vi "Read Key (Variant)__ogtk.vi"(5 "format string (%;%f)":string="%f", 7 "section":string, 8 "error in (no error)":errorcluster, 9 "type":variant, 10 "key (optional)":string, 11 "refnum":T1) -> (0 "error out":errorcluster, 1 "key-value":variant, 2 "found?":bool, 3 "refnum out":T1)   [LabVIEW 2017]
doc: "Reads a value associated with key in a specified section of the configuration data identified by refnum. If \"key\" input is not specified, the name of the variant object is used as the key. the \"found?\" output will be TRUE for compount objects (clusters) only if all elements (recursively) are found.\n\nFor example a Boolean named \"Enable\" with a value of TRUE would correspond to the key-value pair:\n\nEnable=TRUE\n\nNote: Special characters in section and key names will be escape-coded. These include the following: \\00-\\1F (non-printable chars); \"[\", \"]\", and \"=\" (INI syntax elements); \\FE (\"þ\") and \\FF (\"ÿ\") (legacy bracket encoding); Additionally, the escape character, \"\\\", will be escaped as \"\\\\\"."
uses:
  <vilib>/Utility/config.llb/Config Data RefNum.ctl
  <vilib>/Utility/config.llb/Read Key (String).vi
  <vilib>/Utility/config.llb/Read Key (Path).vi
  <vilib>/Utility/config.llb/Read Key (Boolean).vi
  <vilib>/Utility/config.llb/Read Key (Double).vi
  <vilib>/Utility/config.llb/Read Key (U32).vi
  <vilib>/Utility/config.llb/Read Key (I32).vi
  <vilib>/Utility/config.llb/NI_LVConfig.lvlib
panel:
  in  "Ref for recursive call":refnum<vi>
  # "Read Key (Variant).vi\n\nReads a variant key-value from INI file.\n\nPlease visit http://www.OpenG.org to learn about the\nOpen Source LabVIEW software movement.\n\nNOTICE -- YOU MUST LEAVE THIS NOTICE IN PLACE.  PER THE TERMS OF THE LICENSE BELOW, YOU MAY SUBLICENSE THIS SOFTWARE \nIN ANY WAY THAT DOES NOT CONFLICT WITH THIS LICENSE.\n\n### BSD License (http://www.opensource.org/licenses/bsd-license.php) Begin ###\n \nCopyright (c) 2002, Jean-Pierre Drolet <drolet_jp@hotmail.com>\nCopyright (c) 2002-2006, Jim Kring <jim@jimkring.com>\n\nAll rights reserved.\n\nRedistribution and use in source and binary forms, with or without modification, are permitted provided that the following conditions are met:\n\n    * Redistributions of source code must retain the above copyright notice, this list of conditions and the following disclaimer.\n    * Redistributions in binary form must reproduce the above copyright notice, this list of conditions and the following disclaimer in the \n       documentation and/or other materials provided with the distribution.\n    * Neither the name of SciWare, James Kring, Inc., nor the names of its contributors may be used to endorse or promote products derived \n       from this software without specific prior written permission.\n\nTHIS SOFTWARE IS PROVIDED BY THE COPYRIGHT HOLDERS AND CONTRIBUTORS \"AS IS\" AND ANY EXPRESS OR IMPLIED WARRANTIES, \nINCLUDING, BUT NOT LIMITED TO, THE IMPLIED WARRANTIES OF MERCHANTABILITY AND FITNESS FOR A PARTICULAR PURPOSE ARE \nDISCLAIMED. IN NO EVENT SHALL THE COPYRIGHT OWNER OR CONTRIBUTORS BE LIABLE FOR ANY DIRECT, INDIRECT, INCIDENTAL,\n SPECIAL, EXEMPLARY, OR CONSEQUENTIAL DAMAGES (INCLUDING, BUT NOT LIMITED TO, PROCUREMENT OF SUBSTITUTE GOODS OR \nSERVICES; LOSS OF USE, DATA, OR PROFITS; OR BUSINESS INTERRUPTION) HOWEVER CAUSED AND ON ANY THEORY OF LIABILITY, \nWHETHER IN CONTRACT, STRICT LIABILITY, OR TORT (INCLUDING NEGLIGENCE OR OTHERWISE) ARISING IN ANY WAY OUT OF THE USE \nOF THIS SOFTWARE, EVEN IF ADVISED OF THE POSSIBILITY OF SUCH DAMAGE.\n\n### BSD License End ###"
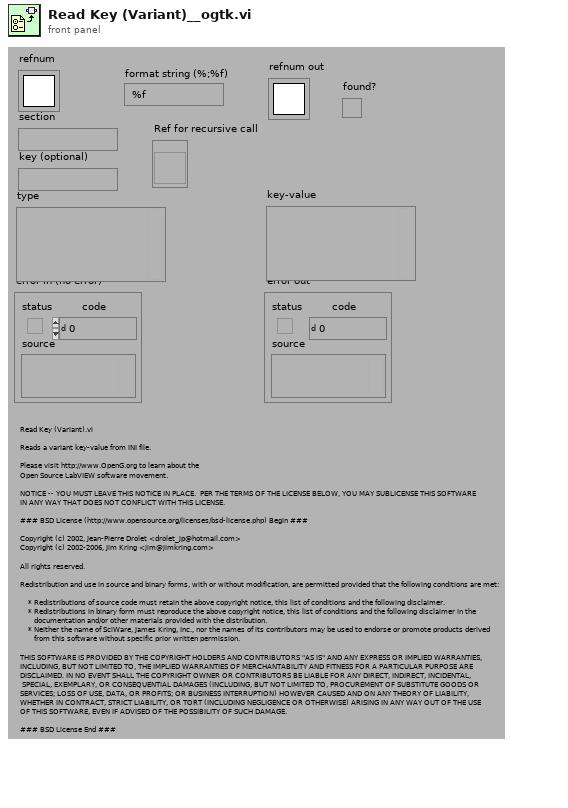
[diagram p1: front panel]
types:
  T1 = typedef "NI_LVConfig.lvlib/Config Data RefNum.ctl" = refnum<k1>
  T2 = typedef "Type Descriptor Enumeration__ogtk.ctl" = enum8{"<Null>", "I8", "I16", "I32", "I64", "U8", "U16", "U32", "U64", "SGL", "DBL", "EXT", "CSG", "CDB", "CXT", "0x0F", "0x10", "0x11", "0x12", "0x13", "0x14", "Enum U8", "Enum U16", "Enum U32", "Enum U64", "SGL PQ", "DBL PQ", "EXT PQ", "CSG PQ", "CDB PQ", "CXT PQ", "0x1F", "0x20", "Boolean", "0x22", "0x23", "0x24", "0x25", "0x26", "0x27", "0x28", "0x29", "0x2A", "0x2B", "0x2C", "0x2D", "0x2E", "0x2F", "String", "0x31", "Path", "Pict", "0x34", "0x35", "0x36", "DAQ", "0x38", "0x39", "0x3A", "0x3B", "0x3C", "0x3D", "0x3E", "0x3F", "Array", "0x41", "0x42", "0x43", "0x44", "0x45", "0x46", "0x47", "0x48", "0x49", "0x4A", "0x4B", "0x4C", "0x4D", "0x4E", "0x4F", "Cluster", "0x51", "0x52", "Variant", "Waveform", "0x55", "0x56", "0x57", "0x58", "0x59", "0x5A", "0x5B", "0x5C", "0x5D", "0x5E", "0x5F", "0x60", "0x61", "0x62", "0x63", "0x64", "0x65", "0x66", "0x67", "0x68", "0x69", "0x6A", "0x6B", "0x6C", "0x6D", "0x6E", "0x6F", "Refnum"}
  T3 = typedef "Type Descriptor__ogtk.ctl" = i16[]
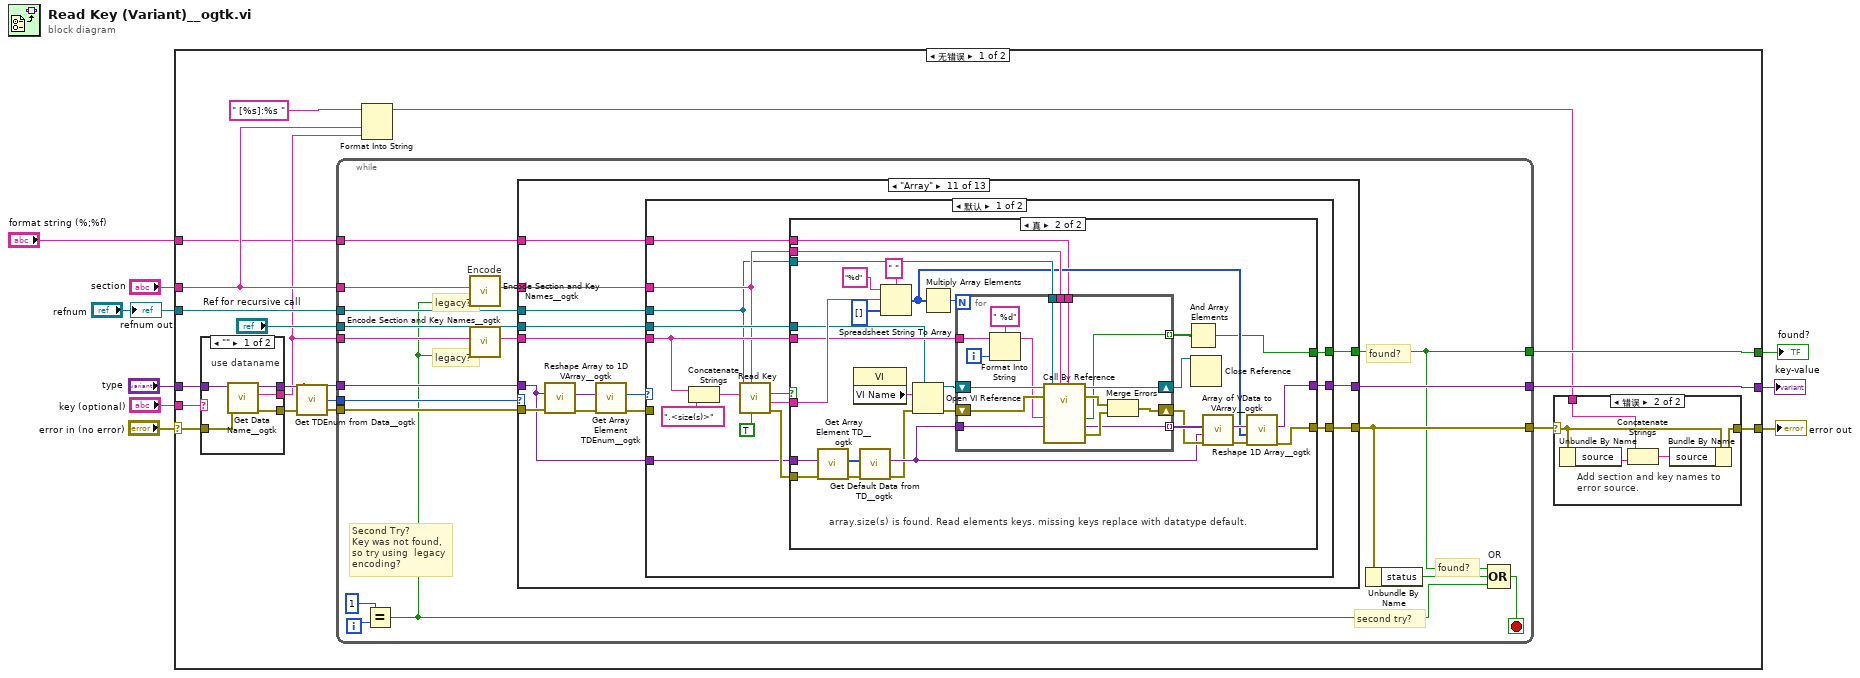
[diagram p0: block diagram]
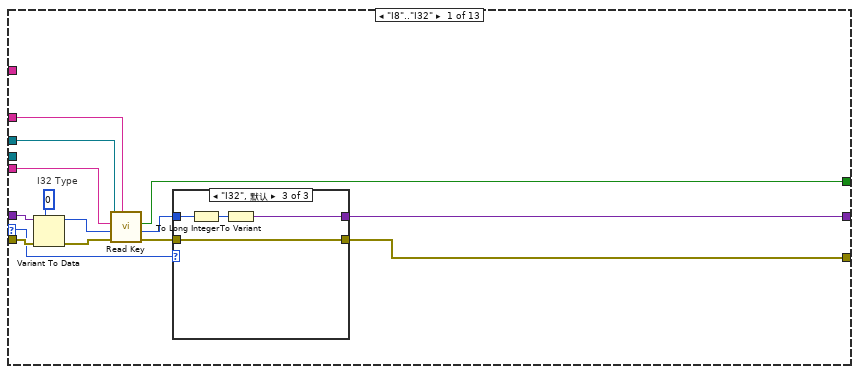
[diagram p2: hidden frame]
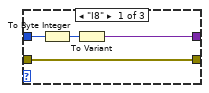
[diagram p3: hidden frame]
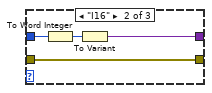
[diagram p4: hidden frame]
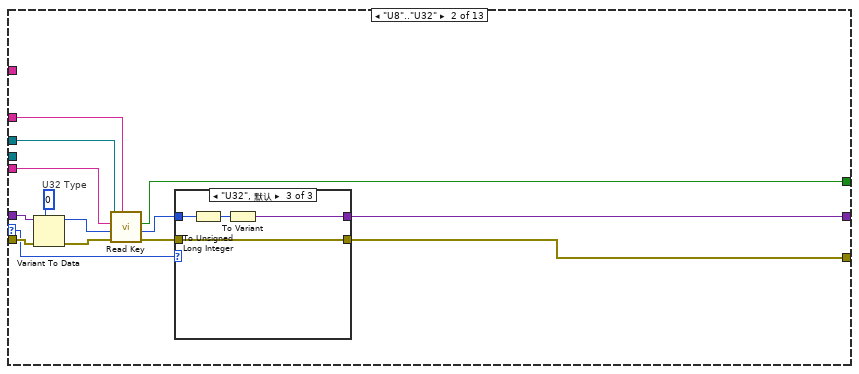
[diagram p5: hidden frame]
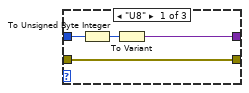
[diagram p6: hidden frame]
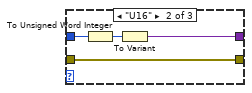
[diagram p7: hidden frame]
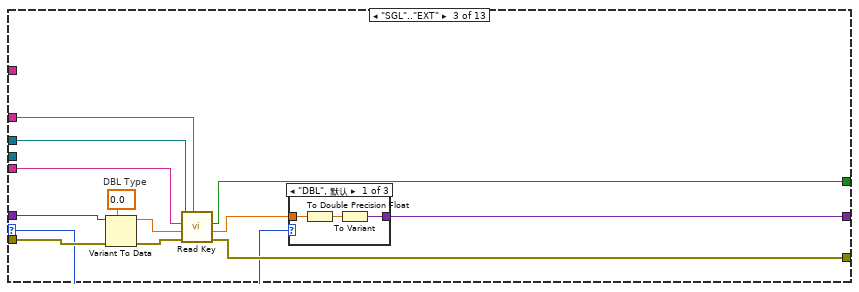
[diagram p8: hidden frame]
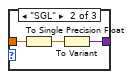
[diagram p9: hidden frame]
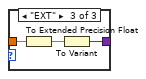
[diagram p10: hidden frame]
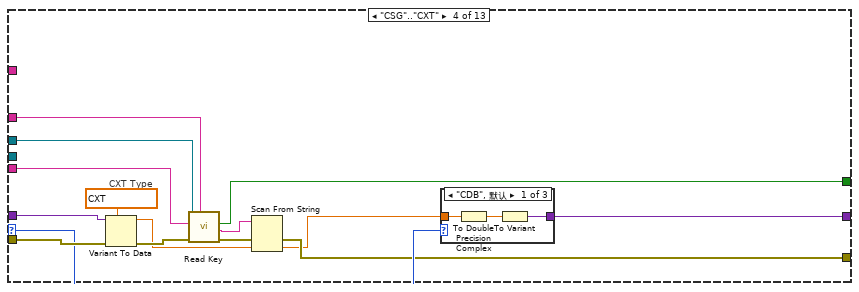
[diagram p11: hidden frame]
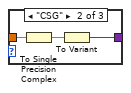
[diagram p12: hidden frame]
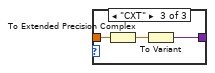
[diagram p13: hidden frame]
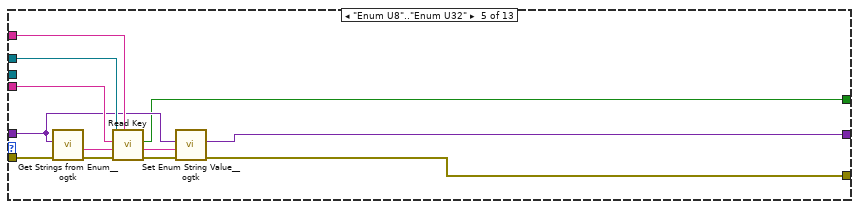
[diagram p14: hidden frame]
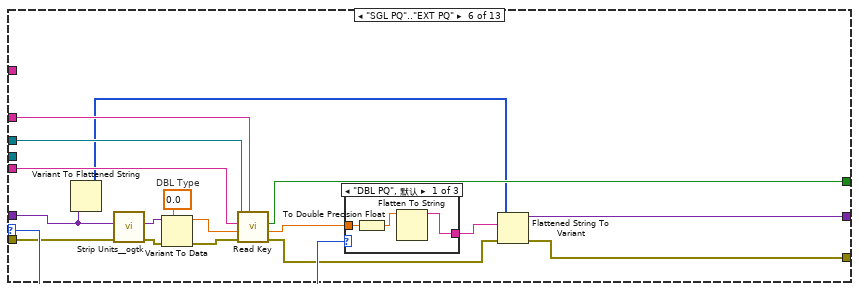
[diagram p15: hidden frame]
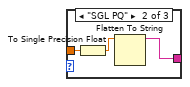
[diagram p16: hidden frame]
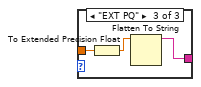
[diagram p17: hidden frame]
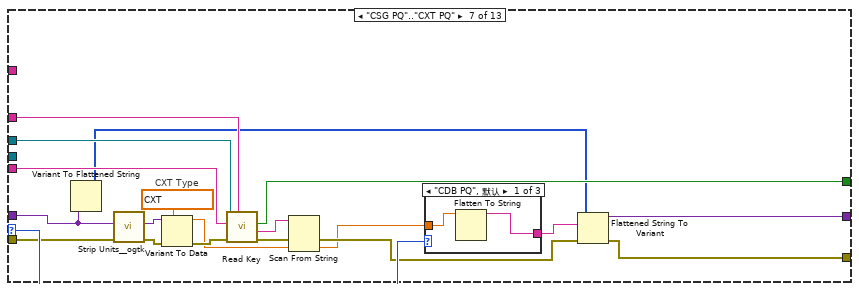
[diagram p18: hidden frame]
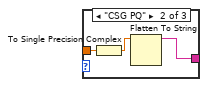
[diagram p19: hidden frame]
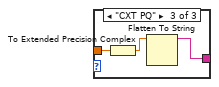
[diagram p20: hidden frame]
diagram:
  n1 = case shown="无错误" "error in (no error)" {
    selector: "error in (no error)" -> [w21 w464]
    tunnel: "refnum" -> [w25 _]
    tunnel: [w15 w464] -> w9
    tunnel: "type" -> [w23 _]
    tunnel: "key (optional)" -> [w22 _]
    tunnel: "section" -> [w12 _]
    tunnel: [w24 variant ("Variant")] -> w4
    tunnel: [w18 FALSE ("found?")] -> w2
    tunnel: "format string (%;%f)" -> [w10 _]
    frame No Error {
      n2 = case shown="\"\"" w22 {
        selector: w22 -> [_ w461]
        tunnel: [w458 w461] -> w11
        tunnel: w23 -> [w455 w459]
        tunnel: w21 -> [w457 w460]
        tunnel: [w456 w460] -> w20
        tunnel: [w454 w459] -> w19
        frame "" {
          # "use dataname"
          n3 = call "Get Data Name__ogtk.vi"("error in (no error)"=w457, "Data"=w455) -> ("error out"=w456:errorcluster, "Data Name"=w458:string, "Data dup"=w454:variant)  [unwired: 7 in]
        }
        frame Default {
          # "use optional\nkey"
        }
      }
      n4 = call "Get TDEnum from Data__ogtk.vi"("Data"=w19) -> ("Type Descriptor Enumeration"=w26:T2)  [unwired: 4 in]
      n5 = while {
        tunnel: w26 -> [w44]
        tunnel: w25 -> [w43]
        tunnel: [w42] -> w24
        tunnel: w20 -> [w41]
        tunnel: w19 -> [w40]
        tunnel: [w32] -> w18
        tunnel: "Ref for recursive call" -> [w39]
        tunnel: [w34] -> w16
        tunnel: w12 -> [w37]
        tunnel: w11 -> [w36]
        tunnel: w10 -> [w27]
        i -> [w31]
        stop <- w29 stop-if-true
        # "found?"
        # "found?"
        # "second try?"
        # "legacy?"
        # "legacy?"
        # "Second Try?\nKey was not found, so try using  legacy encoding?"
        # "Encode"
        n6 = Equal?(x=1, y=w31) -> (x = y?=w28:bool)
        n7 = call "Encode Section and Key Names__ogtk.vi"("use legacy encoding scheme? (FALSE)"=w28, "string"=w37) -> ("encoded string"=w38:string)  [unwired: 9 in]
        n8 = call "Encode Section and Key Names__ogtk.vi"("use legacy encoding scheme? (FALSE)"=w28, "string"=w36) -> ("encoded string"=w35:string)  [unwired: 9 in]
        n9 = case shown="\"Array\"" w44 {
          selector: w44 -> [w47 w73 w97 w124 _ w164 w195 _ _ _ _ _ _]
          tunnel: w40 -> [w57 w83 w108 w132 w145 w157 w189 w220 w232 w244 w248 w395 w444]
          tunnel: w43 -> [w56 w82 w107 w131 w154 w171 w200 w219 w231 w243 w255 w409 w447]
          tunnel: [w46 w71 w105 w122 w147 w159 w191 w217 w229 w241 w252 w398 w438] -> w34
          tunnel: w41 -> [w54 w80 w104 w129 w151 w163 w194 w216 w228 w240 w258 w397 w440]
          tunnel: w35 -> [w53 w79 w103 w128 w153 w169 w198 w215 w227 w239 w249 w407 w446]
          tunnel: w38 -> [w52 w78 w102 w127 w152 w168 w197 w214 w226 w238 w250 w408 w445]
          tunnel: [w45 w75 w99 w126 w144 w155 w187 w211 w225 w235 w253 w399 w441] -> w42
          tunnel: [w50 w74 w98 w125 w143 w165 w196 w210 w222 w234 w251 w403 w436] -> w32
          tunnel: w39 -> [_ _ _ _ _ _ _ _ _ _ w254 w402 _]
          tunnel: w27 -> [_ _ _ _ _ _ _ _ _ _ w246 w392 _]
          frame "I8".."I32" {
            # "I32 Type"
            n10 = Variant To Data(error in=w54, type=0, Variant=w57) -> (data=w51:i32, error out=w55:errorcluster)
            n11 = call-poly <vilib>:"Read Key.vi"("section"=w52, "error in (no error)"=w55, "default value"=w51, "key"=w53, "refnum"=w56) -> ("error out"=w49:errorcluster, "value"=w48:i32, "found?"=w50:bool)  [unwired: 3 in, 1 out]
            n12 = case shown="\"I32\", 默认" w47 {
              tunnel: w48 -> [w62 w66 w70]
              tunnel: [w61 w65 w69] -> w45
              tunnel: w49 -> [w59 w63 w67]
              tunnel: [w59 w63 w67] -> w46
              frame "I8" {
                n13 = To Byte Integer(number=w62) -> (8bit integer=w60:i8)
                n14 = To Variant(anything=w60) -> (Variant=w61:variant)
              }
              frame "I16" {
                n15 = To Word Integer(number=w66) -> (16bit integer=w64:i16)
                n16 = To Variant(anything=w64) -> (Variant=w65:variant)
              }
              frame "I32", Default {
                n17 = To Long Integer(number=w70) -> (32bit integer=w68:i32)
                n18 = To Variant(anything=w68) -> (Variant=w69:variant)
              }
            }
          }
          frame "U8".."U32" {
            # "U32 Type"
            n19 = Variant To Data(error in=w80, type=u32 0, Variant=w83) -> (data=w77:u32, error out=w81:errorcluster)
            n20 = call-poly <vilib>:"Read Key.vi"("section"=w78, "error in (no error)"=w81, "default value"=w77, "key"=w79, "refnum"=w82) -> ("error out"=w72:errorcluster, "value"=w76:u32, "found?"=w74:bool)  [unwired: 3 in, 1 out]
            n21 = case shown="\"U32\", 默认" w73 {
              tunnel: w76 -> [w88 w92 w96]
              tunnel: [w87 w91 w95] -> w75
              tunnel: w72 -> [w85 w89 w93]
              tunnel: [w85 w89 w93] -> w71
              frame "U8" {
                n22 = To Unsigned Byte Integer(number=w88) -> (unsigned 8bit integer=w86:u8)
                n23 = To Variant(anything=w86) -> (Variant=w87:variant)
              }
              frame "U16" {
                n24 = To Unsigned Word Integer(number=w92) -> (unsigned 16bit integer=w90:u16)
                n25 = To Variant(anything=w90) -> (Variant=w91:variant)
              }
              frame "U32", Default {
                n26 = To Unsigned Long Integer(number=w96) -> (unsigned 32bit integer=w94:u32)
                n27 = To Variant(anything=w94) -> (Variant=w95:variant)
              }
            }
          }
          frame "SGL".."EXT" {
            # "DBL Type"
            n28 = Variant To Data(error in=w104, type=0.0, Variant=w108) -> (data=w101:dbl, error out=w106:errorcluster)
            n29 = call-poly <vilib>:"Read Key.vi"("section"=w102, "error in (no error)"=w106, "default value"=w101, "key"=w103, "refnum"=w107) -> ("error out"=w105:errorcluster, "value"=w100:dbl, "found?"=w98:bool)  [unwired: 3 in, 1 out]
            n30 = case shown="\"DBL\", 默认" w97 {
              tunnel: w100 -> [w112 w115 w118]
              tunnel: [w111 w114 w117] -> w99
              frame "DBL", Default {
                n31 = To Double Precision Float(number=w112) -> (double precision float=w110:dbl)
                n32 = To Variant(anything=w110) -> (Variant=w111:variant)
              }
              frame "SGL" {
                n33 = To Single Precision Float(number=w115) -> (single precision float=w113:sgl)
                n34 = To Variant(anything=w113) -> (Variant=w114:variant)
              }
              frame "EXT" {
                n35 = To Extended Precision Float(1:w118) -> (0:w116:ext)
                n36 = To Variant(anything=w116) -> (Variant=w117:variant)
              }
            }
          }
          frame "CSG".."CXT" {
            # "CXT Type"
            n37 = Variant To Data(error in=w129, type=cxt 0.0+0.0i, Variant=w132) -> (data=w120:cxt, error out=w130:errorcluster)
            n38 = call-poly <vilib>:"Read Key.vi"("section"=w127, "error in (no error)"=w130, "key"=w128, "refnum"=w131) -> ("error out"=w123:errorcluster, "value"=w121:string, "found?"=w125:bool)  [unwired: 4 in, 1 out]
            n39 = Scan From String(input string=w121, error in=w123, default 1=w120) -> (error out=w122:errorcluster, output 1=w119:cxt)  [unwired: 2 in, 2 out]
            n40 = case shown="\"CDB\", 默认" w124 {
              tunnel: w119 -> [w136 w139 w142]
              tunnel: [w135 w138 w141] -> w126
              frame "CDB", Default {
                n41 = To Double Precision Complex(1:w136) -> (0:w134:cdb)
                n42 = To Variant(anything=w134) -> (Variant=w135:variant)
              }
              frame "CSG" {
                n43 = To Single Precision Complex(1:w139) -> (0:w137:csg)
                n44 = To Variant(anything=w137) -> (Variant=w138:variant)
              }
              frame "CXT" {
                n45 = To Extended Precision Complex(1:w142) -> (0:w140:cxt)
                n46 = To Variant(anything=w140) -> (Variant=w141:variant)
              }
            }
          }
          frame "Enum U8".."Enum U32" {
            n47 = call "Get Strings from Enum__ogtk.vi"("error in (no error)"=w151, "Enum"=w145) -> ("error out"=w150:errorcluster, "String Value"=w149:string)  [unwired: 6 in, 2 out]
            n48 = call-poly <vilib>:"Read Key.vi"("section"=w152, "error in (no error)"=w150, "default value"=w149, "key"=w153, "refnum"=w154) -> ("error out"=w148:errorcluster, "value"=w146:string, "found?"=w143:bool)  [unwired: 3 in, 1 out]
            n49 = call "Set Enum String Value__ogtk.vi"("error in (no error)"=w148, "String Value"=w146, "Default Enum Value"=w145) -> ("error out"=w147:errorcluster, "Enum"=w144:variant)  [unwired: 7 in]
          }
          frame "SGL PQ".."EXT PQ" {
            # "DBL Type"
            n50 = Variant To Flattened String(Variant=w157) -> (1:w156:i16[])  [unwired: 1 out]
            n51 = call "Strip Units__ogtk.vi"("error in (no error)"=w163, "Number or 1D array with units"=w157) -> ("error out"=w161:errorcluster, "Pure Number(s) (base units)"=w162:variant)  [unwired: 8 in]
            n52 = Variant To Data(error in=w161, type=0.0, Variant=w162) -> (data=w167:dbl, error out=w170:errorcluster)
            n53 = call-poly <vilib>:"Read Key.vi"("section"=w168, "error in (no error)"=w170, "default value"=w167, "key"=w169, "refnum"=w171) -> ("error out"=w160:errorcluster, "value"=w166:dbl, "found?"=w165:bool)  [unwired: 3 in, 1 out]
            n54 = case shown="\"DBL PQ\", 默认" w164 {
              tunnel: w166 -> [w175 w178 w181]
              tunnel: [w174 w176 w179] -> w158
              frame "DBL PQ", Default {
                n55 = To Double Precision Float(number=w175) -> (double precision float=w173:dbl)
                n56 = Flatten To String(anything=w173) -> (data string=w174:string)  [unwired: 3 in, 2 out]
              }
              frame "SGL PQ" {
                n57 = To Single Precision Float(number=w178) -> (single precision float=w177:sgl)
                n58 = Flatten To String(anything=w177) -> (data string=w176:string)  [unwired: 3 in, 2 out]
              }
              frame "EXT PQ" {
                n59 = To Extended Precision Float(1:w181) -> (0:w180:ext)
                n60 = Flatten To String(anything=w180) -> (data string=w179:string)  [unwired: 3 in, 2 out]
              }
            }
            n61 = Flattened String To Variant(4:w160, 6:w158, 7:w156) -> (0:w159:errorcluster, 3:w155:variant)
          }
          frame "CSG PQ".."CXT PQ" {
            # "CXT Type"
            n62 = Variant To Flattened String(Variant=w189) -> (1:w188:i16[])  [unwired: 1 out]
            n63 = call "Strip Units__ogtk.vi"("error in (no error)"=w194, "Number or 1D array with units"=w189) -> ("error out"=w192:errorcluster, "Pure Number(s) (base units)"=w193:variant)  [unwired: 8 in]
            n64 = Variant To Data(error in=w192, type=cxt 0.0+0.0i, Variant=w193) -> (data=w183:cxt, error out=w199:errorcluster)
            n65 = call-poly <vilib>:"Read Key.vi"("section"=w197, "error in (no error)"=w199, "key"=w198, "refnum"=w200) -> ("error out"=w185:errorcluster, "value"=w184:string, "found?"=w196:bool)  [unwired: 4 in, 1 out]
            n66 = Scan From String(input string=w184, error in=w185, default 1=w183) -> (error out=w186:errorcluster, output 1=w182:cxt)  [unwired: 2 in, 2 out]
            n67 = case shown="\"CDB PQ\", 默认" w195 {
              tunnel: w182 -> [w203 w206 w209]
              tunnel: [w202 w204 w207] -> w190
              frame "CDB PQ", Default {
                n68 = Flatten To String(anything=w203) -> (data string=w202:string)  [unwired: 3 in, 2 out]
              }
              frame "CSG PQ" {
                n69 = To Single Precision Complex(1:w206) -> (0:w205:csg)
                n70 = Flatten To String(anything=w205) -> (data string=w204:string)  [unwired: 3 in, 2 out]
              }
              frame "CXT PQ" {
                n71 = To Extended Precision Complex(1:w209) -> (0:w208:cxt)
                n72 = Flatten To String(anything=w208) -> (data string=w207:string)  [unwired: 3 in, 2 out]
              }
            }
            n73 = Flattened String To Variant(4:w186, 6:w190, 7:w188) -> (0:w191:errorcluster, 3:w187:variant)
          }
          frame "Boolean" {
            # "Boolean Type"
            n74 = Variant To Data(error in=w216, type=FALSE, Variant=w220) -> (data=w213:bool, error out=w218:errorcluster)
            n75 = call-poly <vilib>:"Read Key.vi"("section"=w214, "error in (no error)"=w218, "default value"=w213, "key"=w215, "refnum"=w219) -> ("error out"=w217:errorcluster, "value"=w212:bool, "found?"=w210:bool)  [unwired: 3 in, 1 out]
            n76 = To Variant(anything=w212) -> (Variant=w211:variant)
          }
          frame "String", "DAQ" {
            # "String Type"
            n77 = Variant To Data(error in=w228, type="", Variant=w232) -> (data=w223:string, error out=w230:errorcluster)
            n78 = call-poly <vilib>:"Read Key.vi"("section"=w226, "error in (no error)"=w230, "default value"=w223, "key"=w227, "refnum"=w231) -> ("error out"=w229:errorcluster, "value"=w224:string, "found?"=w222:bool)  [unwired: 3 in, 1 out]
            n79 = To Variant(anything=w224) -> (Variant=w225:variant)
          }
          frame "Path" {
            # "Path Type"
            n80 = Variant To Data(error in=w240, type=path "", Variant=w244) -> (data=w237:path, error out=w242:errorcluster)
            n81 = call-poly <vilib>:"Read Key.vi"("section"=w238, "error in (no error)"=w242, "default value"=w237, "key"=w239, "refnum"=w243) -> ("error out"=w241:errorcluster, "value"=w236:path, "found?"=w234:bool)  [unwired: 3 in, 1 out]
            n82 = To Variant(anything=w236) -> (Variant=w235:variant)
          }
          frame "Array" {
            n83 = call "Reshape Array to 1D VArray__ogtk.vi"("error in (no error)"=w258, "MultiD Array"=w248) -> ("error out"=w259:errorcluster, "1D VArray"=w247:variant)  [unwired: 7 in, 1 out]
            n84 = call "Get Array Element TDEnum__ogtk.vi"("error in (no error)"=w259, "Array"=w247) -> ("error out"=w256:errorcluster, "Element Type"=w257:T2)  [unwired: 8 in]
            n85 = case shown="默认" w257 {
              selector: w257 -> [_ w338]
              tunnel: w256 -> [_ w348]
              tunnel: w248 -> [w269 w326]
              tunnel: w250 -> [w267 w349]
              tunnel: w255 -> [w266 w350]
              tunnel: w249 -> [w270 w351]
              tunnel: w254 -> [w268 _]
              tunnel: [w264 w325] -> w253
              tunnel: [w263 errorcluster {"status"=FALSE, "code"=0, "source"=""} ("error out")] -> w252
              tunnel: [w262 w347] -> w251
              tunnel: w246 -> [w260 w323]
              frame Default {
                n86 = Concatenate Strings(w270, ".<size(s)>" ("Substring")) -> (w273:string)
                n87 = call-poly <vilib>:"Read Key.vi"("read raw string? (F)"=TRUE, "section"=w267, "key"=w273, "refnum"=w266) -> ("error out"=w271:errorcluster, "value"=w272:string, "found?"=w261:bool)  [unwired: 4 in, 1 out]
                n88 = case shown="真" w261 {
                  tunnel: w272 -> [_ w304]
                  tunnel: w271 -> [_ w280]
                  tunnel: w270 -> [_ w299]
                  tunnel: w269 -> [w276 w298]
                  tunnel: w268 -> [_ w297]
                  tunnel: w267 -> [_ w295]
                  tunnel: w266 -> [_ w294]
                  tunnel: [w276 w287] -> w264
                  tunnel: [errorcluster {"status"=FALSE, "code"=0, "source"=""} ("error out") w286] -> w263
                  tunnel: [FALSE w284] -> w262
                  tunnel: w260 -> [_ w278]
                  frame False {
                    # "array size(s) not found. Ignore element keys (if any) and return input array"
                  }
                  frame True {
                    # "array.size(s) is found. Read elements keys. missing keys replace with datatype default."
                    n89 = call "Get Array Element TD__ogtk.vi"("error in (no error)"=w280, "Array"=w298) -> ("error out"=w282:errorcluster, "Type Descriptor"=w283:T3)  [unwired: 8 in]
                    n90 = property class="VI"() -> ("VI Name"=w301:string)  [unwired: 2 in, 2 out]
                    n91 = call "Get Default Data from TD__ogtk.vi"("error in (no error)"=w282, "Type Descriptor"=w283) -> ("error out"=w279:errorcluster, "Default VData"=w281:variant)  [unwired: 8 in]
                    n92 = Spreadsheet String To Array(delimiter (Tab)=" ", format string="%d", spreadsheet string=w304, array type (2D Dbl)=u32[] [] ("Array Constant")) -> (array=w288:u32[])
                    n93 = Open VI Reference(type specifier VI Refnum (for type only)=w297, vi path=w301, error in (no error)=w279) -> (vi reference=w296:refnum<vi>, error out=w300:errorcluster)  [unwired: 3 in]
                    n94 = Multiply Array Elements(1:w288) -> (0:w302:u32)
                    n95 = for {
                      N: w302 -> [_]
                      shift-right: [w316] -> w291
                      shift-left: w300 -> [w313]
                      shift-right: [w317] -> w293
                      shift-left: w296 -> [w315]
                      tunnel: w299 -> [w320]
                      tunnel: w281 -> [w314]
                      tunnel: w295 -> [w311]
                      tunnel: w294 -> [w310]
                      tunnel: [w309] -> w292 mode=indexing
                      tunnel: [w308] -> w285 mode=indexing
                      tunnel: w278 -> [w307]
                      i -> [w321]
                      n96 = Format Into String(format string=" %d" ("Format String"), initial string=w320, w321) -> (resulting string=w312:string)  [unwired: 1 in, 1 out]
                      n97 = call-by-ref "?"(reference=w315, error in=w313, "format string (%;%f"=w307, "section"=w311, "type"=w314, "key (optional)"=w312, "refnum"=w310) -> (reference out=w317:refnum<vi>, error out=w319:errorcluster, "error out"=w318:errorcluster, "key-value"=w309:variant, "found?"=w308:bool)  [unwired: 3 in, 1 out]
                      n98 = Merge Errors(w319, w318) -> (w316:errorcluster)
                    }
                    n99 = And Array Elements(Boolean array=w285) -> (logical AND=w284:bool)
                    n100 = Close Reference(reference=w293) -> ()  [unwired: 1 in, 1 out]
                    n101 = call "Array of VData to VArray__ogtk.vi"("error in (no error)"=w291, "Element Type (when empty)"=w281, "1D Array of VData"=w292) -> ("error out"=w290:errorcluster, "VArray"=w289:variant)  [unwired: 7 in]
                    n102 = call "Reshape 1D Array__ogtk.vi"("error in (no error)"=w290, "Size(s)"=w288, "1D Array"=w289) -> ("error out"=w286:errorcluster, "Reshaped VArray"=w287:variant)  [unwired: 7 in]
                  }
                }
              }
              frame "I8".."I32", "U8".."U32", "SGL".."EXT", "SGL PQ".."EXT PQ" {
                n103 = call-poly <vilib>:"Read Key.vi"("section"=w349, "error in (no error)"=w348, "key"=w351, "refnum"=w350) -> ("error out"=w346:errorcluster, "value"=w352:string, "found?"=w347:bool)  [unwired: 4 in, 1 out]
                n104 = Scan From String(format string="<size(s)=%[\\s0-9]> " ("regular expression"), input string=w352, error in=w346) -> (remaining string=w339:string, error out=w329:errorcluster, output 1=w344:string)  [unwired: 2 in, 1 out]
                n105 = Variant To Flattened String(Variant=w326) -> (data string=w331:string, 1:w332:i16[])
                n106 = Spreadsheet String To Array(delimiter (Tab)=" ", format string="%d", spreadsheet string=w344, array type (2D Dbl)=u32[] []) -> (array=w345:u32[])
                n107 = Type Cast(x=w345) -> (*(type *) &x=w336:string)  [unwired: 1 in]
                n108 = Spreadsheet String To Array(delimiter (Tab)=" ", format string=w323, spreadsheet string=w339, array type (2D Dbl)=dbl[] []) -> (array=w337:dbl[])
                n109 = case shown="\"SGL\", \"SGL PQ\"" w338 {
                  tunnel: w337 -> [_ w359 w363 w367 w371 w375 w379 w383 w385 w389]
                  tunnel: [w354 w357 w361 w365 w369 w373 w377 w381 w387 w391] -> w334
                  tunnel: ["" w356 w360 w364 w368 w372 w376 w380 w386 w390] -> w333
                  tunnel: w336 -> [_ w356 w360 w364 w368 w372 w376 w380 w386 w390]
                  tunnel: w331 -> [w354 _ _ _ _ _ _ _ _ _]
                  frame Default {
                  }
                  frame "I8" {
                    n110 = To Byte Integer(number=w359) -> (8bit integer=w358:i8[])
                    n111 = Type Cast(x=w358) -> (*(type *) &x=w357:string)  [unwired: 1 in]
                  }
                  frame "I16" {
                    n112 = To Word Integer(number=w363) -> (16bit integer=w362:i16[])
                    n113 = Type Cast(x=w362) -> (*(type *) &x=w361:string)  [unwired: 1 in]
                  }
                  frame "I32" {
                    n114 = To Long Integer(number=w367) -> (32bit integer=w366:i32[])
                    n115 = Type Cast(x=w366) -> (*(type *) &x=w365:string)  [unwired: 1 in]
                  }
                  frame "U8" {
                    n116 = To Unsigned Byte Integer(number=w371) -> (unsigned 8bit integer=w370:u8[])
                    n117 = Type Cast(x=w370) -> (*(type *) &x=w369:string)  [unwired: 1 in]
                  }
                  frame "U16" {
                    n118 = To Unsigned Word Integer(number=w375) -> (unsigned 16bit integer=w374:u16[])
                    n119 = Type Cast(x=w374) -> (*(type *) &x=w373:string)  [unwired: 1 in]
                  }
                  frame "U32" {
                    n120 = To Unsigned Long Integer(number=w379) -> (unsigned 32bit integer=w378:u32[])
                    n121 = Type Cast(x=w378) -> (*(type *) &x=w377:string)  [unwired: 1 in]
                  }
                  frame "SGL", "SGL PQ" {
                    n122 = To Single Precision Float(number=w383) -> (single precision float=w382:sgl[])
                    n123 = Type Cast(x=w382) -> (*(type *) &x=w381:string)  [unwired: 1 in]
                  }
                  frame "DBL", "DBL PQ" {
                    n124 = To Double Precision Float(number=w385) -> (double precision float=w384:dbl[])
                    n125 = Type Cast(x=w384) -> (*(type *) &x=w387:string)  [unwired: 1 in]
                  }
                  frame "EXT", "EXT PQ" {
                    n126 = To Extended Precision Float(1:w389) -> (0:w388:ext[])
                    n127 = Type Cast(x=w388) -> (*(type *) &x=w391:string)  [unwired: 1 in]
                  }
                }
                n128 = Concatenate Strings(w333, w334) -> (w335:string)
                n129 = Flattened String To Variant(4:w329, 6:w335, 7:w332) -> (0:w328:errorcluster, 3:w327:variant)
                n130 = Select(t=w326, s=w328, f=w327) -> (s? t:f=w325:variant)
              }
            }
          }
          frame "Cluster" {
            # ">> Cluster Name >>"
            # "Expand cluster to its elements\nand read keys recursively."
            n131 = call "Get Data Name__ogtk.vi"("error in (no error)"=w397, "Data"=w395) -> ("error out"=w396:errorcluster, "Data Name"=w393:string, "Data dup"=w394:variant)  [unwired: 7 in]
            n132 = call "Cluster to Array of VData__ogtk.vi"("error in (no error)"=w396, "Cluster"=w394) -> ("error out"=w415:errorcluster, "Array of VData"=w414:variant[])  [unwired: 8 in]
            n133 = property class="VI"() -> ("VI Name"=w413:string)  [unwired: 2 in, 2 out]
            n134 = Open VI Reference(type specifier VI Refnum (for type only)=w402, vi path=w413, error in (no error)=w415) -> (vi reference=w410:refnum<vi>, error out=w412:errorcluster)  [unwired: 3 in]
            n135 = for {
              shift-right: [w434] -> w411
              shift-left: w410 -> [w435]
              shift-right: [w419] -> w405
              shift-left: w412 -> [w430]
              tunnel: w414 -> [w428] mode=indexing
              tunnel: w408 -> [w424]
              tunnel: w409 -> [w425]
              tunnel: w407 -> [w432]
              tunnel: [w421] -> w406 mode=indexing
              tunnel: [w417] -> w404 mode=indexing
              tunnel: w392 -> [w416]
              n136 = call "Get Data Name__ogtk.vi"("error in (no error)"=w430, "Data"=w428) -> ("error out"=w429:errorcluster, "Data Name"=w418:string, "Data dup"=w427:variant)  [unwired: 7 in]
              n137 = Format Into String(format string=".%s" ("Format String"), initial string=w432, w418) -> (resulting string=w426:string)  [unwired: 1 in, 1 out]
              n138 = call-by-ref "?"(reference=w435, error in=w429, "format string (%;%f"=w416, "section"=w424, "type"=w427, "key (optional)"=w426, "refnum"=w425) -> (reference out=w434:refnum<vi>, error out=w433:errorcluster, "error out"=w423:errorcluster, "key-value"=w422:variant, "found?"=w417:bool)  [unwired: 3 in, 1 out]
              n139 = Merge Errors(w433, w423) -> (w420:errorcluster)
              n140 = call "Set Data Name__ogtk.vi"("error in (no error)"=w420, "Data Name"=w418, "Data"=w422) -> ("error out"=w419:errorcluster, "Renamed Data"=w421:variant)  [unwired: 7 in]
            }
            n141 = And Array Elements(Boolean array=w404) -> (logical AND=w403:bool)
            n142 = call "Array of VData to VCluster__ogtk.vi"("error in (no error)"=w405, "Array"=w406) -> ("error out"=w401:errorcluster, "VCluster"=w400:variant)  [unwired: 8 in]
            n143 = Close Reference(reference=w411) -> ()  [unwired: 1 in, 1 out]
            n144 = call "Set Data Name__ogtk.vi"("error in (no error)"=w401, "Data Name"=w393, "Data"=w400) -> ("error out"=w398:errorcluster, "Renamed Data"=w399:variant)  [unwired: 7 in]
          }
          frame Default {
            n145 = Variant To Flattened String(Variant=w444) -> (data string=w443:string, 1:w437:i16[])
            n146 = call-poly <vilib>:"Read Key.vi"("section"=w445, "error in (no error)"=w440, "default value"=w443, "key"=w446, "refnum"=w447) -> ("error out"=w439:errorcluster, "value"=w442:string, "found?"=w436:bool)  [unwired: 3 in, 1 out]
            n147 = Flattened String To Variant(4:w439, 6:w442, 7:w437) -> (0:w438:errorcluster, 3:w441:variant)
          }
        }
        n148 = Unbundle By Name(w34) -> ("status"=w33:bool)
        n149 = Compound Arithmetic op=OR "OR"(w32, w33, w28) -> (w29:bool)
      }
      n150 = Format Into String(format string=" [%s]:%s " ("Format String"), w12, w11) -> (resulting string=w13:string)  [unwired: 2 in, 1 out]
      n151 = case shown="错误" w16 {
        selector: w16 -> [w448 w453]
        tunnel: [w448 w452] -> w15
        tunnel: w13 -> [_ w449]
        frame No Error {
        }
        frame Error {
          # "Add section and key names to\nerror source."
          n152 = Unbundle By Name(w453) -> ("source"=w450:string)
          n153 = Concatenate Strings(w449, w450) -> (w451:string)
          n154 = Bundle By Name(cluster=w453, "source"=w451) -> (w452:errorcluster)
        }
      }
    }
    frame Error {
    }
  }
  "error out" <- w9
  "key-value" <- w4
  "found?" <- w2
  "refnum out" <- "refnum"
